vi "Write constant.vi"(8 "error in (no error)":errorcluster, 10 "constant":u16, 11 "rqcBob in":refnum<class "rqcBob.lvclass">) -> (0 "error out":errorcluster, 3 "rqcBob out":refnum<class "rqcBob.lvclass">)   [LabVIEW 2018, in "rqcBob.lvclass"]
uses:
  rqcBob.lvclass
  Custom Controls/rqcBob Main FPGA interface.ctl
  rqcBob.lvclass/rqcBob.ctl
  <vilib>/Utility/error.llb/Error Cluster From Error Code.vi
  <vilib>/rvi/errors/niLvFpgaAdjustHostInterfaceError.vi
  <vilib>/rvi/interface/nirviReadWriteControl/nirviReadWriteControl.xnode
  NiFpgaLv.dll
  <vilib>/rvi/interface/Simulation/niFpgaSimulationCallBeginRW.vi
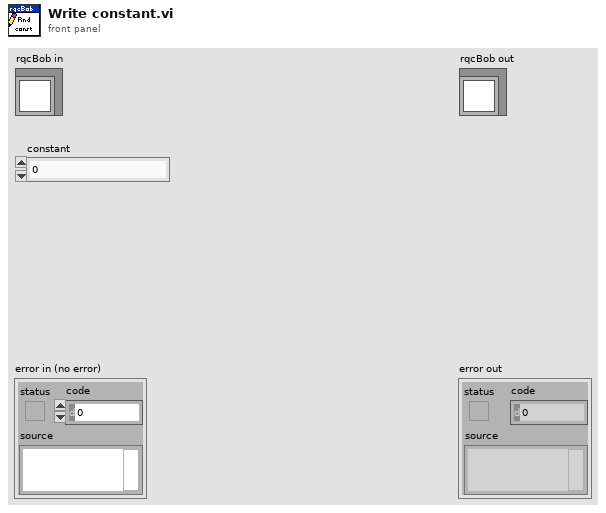
[diagram p1: front panel]
types:
  T1 = typedef "rqcBob.lvclass/rqcBob Main FPGA interface.ctl" = refnum<k20>
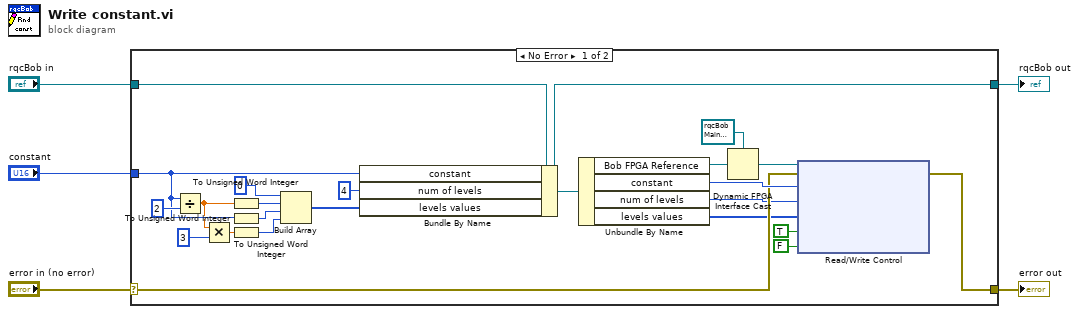
[diagram p0: block diagram]
diagram:
  n1 = case shown="No Error" "error in (no error)" {
    selector: "error in (no error)" -> [w22 w29]
    tunnel: [w21 w29] -> w4
    tunnel: [w23 w30] -> w2
    tunnel: "rqcBob in" -> [w28 w30]
    tunnel: "constant" -> [w13 _]
    frame No Error {
      n2 = Divide(x=w13, y=u16 2) -> (x/y=w12:dbl)
      n3 = Multiply(x=w12, y=u16 3) -> (x*y=w10:dbl)
      n4 = To Unsigned Word Integer(number=w12) -> (unsigned 16bit integer=w17:u16)
      n5 = To Unsigned Word Integer(number=w13) -> (unsigned 16bit integer=w16:u16)
      n6 = To Unsigned Word Integer(number=w10) -> (unsigned 16bit integer=w15:u16)
      n7 = Build Array(u16 0 ("DAC value"), w17, w16, w15) -> (w14:u16[])
      n8 = Bundle By Name(cluster=w28, "constant"=w13, "num of levels"=u16 4 ("rndGen.parameters.num of levels"), "levels values"=w14) -> (w23:refnum<class "rqcBob.lvclass">)
      n9 = Unbundle By Name(w23) -> ("Bob FPGA Reference"=w27:refnum<k20>, "constant"=w24:u16, "num of levels"=w9:u16, "levels values"=w8:u16[])
      n10 = Dynamic FPGA Interface Cast(Session In=T1 refnum ("Bob main FPGA interface"), Type=w27) -> (Session Out=w25:T1)
      n11 = xnode "Read/Write Control"("FPGA VI Reference In"=w25, "error in"=w22, "rndGen.constant"=w24, "rndGen.num of levels"=w9, "rndGen.levels values"=w8, "rndGen.reset"=TRUE, "rndGen.reset"=FALSE) -> ("error out"=w21:errorcluster)  [unwired: 1 out]
    }
    frame Error {
    }
  }
  "error out" <- w4
  "rqcBob out" <- w2
